vi "example_setTerminalPosition.vi"() -> ()   [LabVIEW 2023]
uses:
  <vilib>/Utility/miscctls.llb/LVPositionTypeDef.ctl
  Terminal/Terminal.lvclass
  C:/projects/TLC_Scripto/Source/GObject/GObject.lvclass
  BlockDiagram/Read terminals.vi
  GObject/Read position.vi
  TLC_Scripto.lvlib
  BlockDiagram/BlockDiagram.lvclass
panel:
  out "Array":T1[](array[typedef])
  out "error out":errorcluster
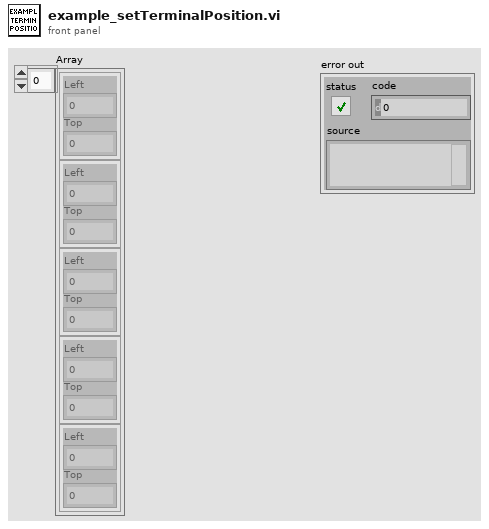
[diagram p1: front panel]
types:
  T1 = typedef "LVPositionTypeDef.ctl" = cluster{"Left":i32, "Top":i32}
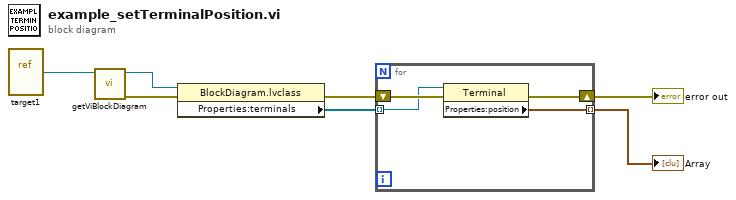
[diagram p0: block diagram]
diagram:
  n1 = vi-ref "target1.vi"() -> (w7:refnum<vi>)
  n2 = call "getViBlockDiagram.vi"("ViRef"=w7) -> ("error out"=w6:errorcluster, "topMostBlockDiagram"=w5:refnum<class "BlockDiagram.lvclass">)  [unwired: 9 in]
  n3 = property class="BlockDiagram.lvclass"(reference=w5, error in=w6) -> (error out=w4:errorcluster, "Properties:terminals"=w3:refnum<class "Terminal.lvclass">[])  [unwired: 1 out]
  n4 = for {
    tunnel: w3 -> [w10] mode=indexing
    tunnel: [w9] -> w2 mode=indexing
    shift-right: [w8] -> w1
    shift-left: w4 -> [w11]
    n5 = property class="Terminal"(reference=w10, error in=w11) -> (error out=w8:errorcluster, "Properties:position"=w9:T1)  [unwired: 1 out]
  }
  "error out" <- w1
  "Array" <- w2
